vi "test Convert Shutdown Furnace to Heater State Enum-Shutdown False.vi"(8 "error in (no error)":errorcluster, 11 "TestCase in":refnum<class "Convert Shutdown Furnace to Heater State Enum.lvclass">) -> (0 "error out":errorcluster, 3 "TestCase out":refnum<class "Convert Shutdown Furnace to Heater State Enum.lvclass">)   [LabVIEW 2018, in "Convert Shutdown Furnace to Heater State Enum.lvclass"]
uses:
  Convert Shutdown Furnace to Heater State Enum.lvclass
  Libraries/Thermal Chamber Controller_DQMH/Heater State--enum.ctl
  Libraries/Thermal Chamber Controller_DQMH/Thermal Chamber Controller_DQMH.lvlib
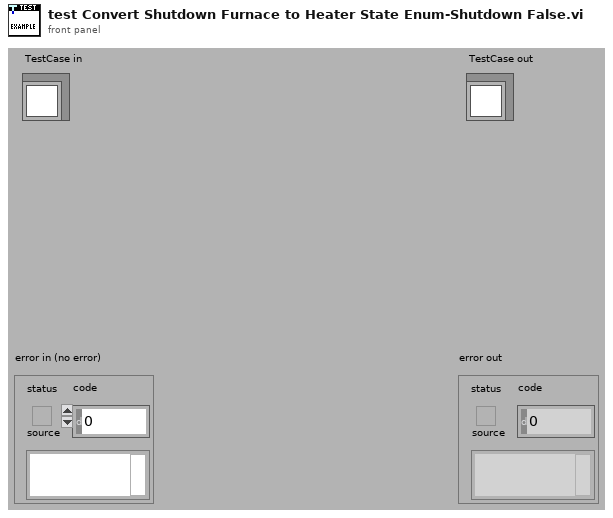
[diagram p1: front panel]
types:
  T1 = typedef "Thermal Chamber Controller_DQMH.lvlib/Heater State--enum.ctl" = enum16{"Heater Enabled", "Heater Disabled"}
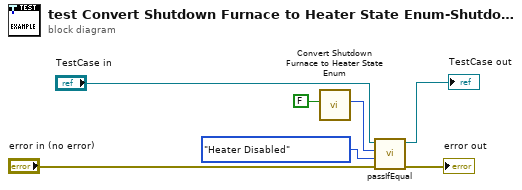
[diagram p0: block diagram]
diagram:
  n1 = call "Convert Shutdown Furnace to Heater State Enum.vi"("Shutdown Furnace?"=FALSE) -> ("Heater State"=w6:T1)  [unwired: 10 in]
  n2 = call-dynamic "passIfEqual.vi"("error in (no error)"="error in (no error)", "y"=Heater_State--enum."Heater Disabled" ("Heater State"), "x"=w6, "TestCase in"="TestCase in") -> ("error out"=→"error out":errorcluster, "TestCase out"=→"TestCase out":refnum<class "Convert Shutdown Furnace to Heater State Enum.lvclass">)  [unwired: 6 in]
